vi "Append To Dataset 1D Double.vi"(8 "Error in (no error)":errorcluster, 10 "data":dbl[](array[numeric]), 11 "Dataset id in":i32) -> (0 "Error out":errorcluster, 3 "Dataset id out":i32)   [LabVIEW 2011]
uses:
  Release/HDF5Tools.dll
  HDF5Tools.lvlib
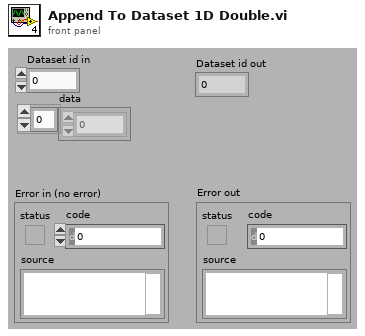
[diagram p1: front panel]
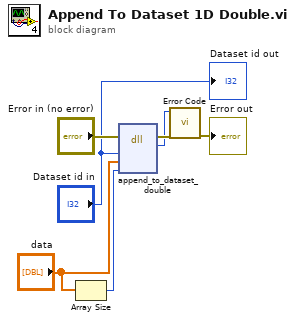
[diagram p0: block diagram]
diagram:
  n1 = Array Size(array="data") -> (size(s)=w2:i32)
  n2 = dll-call lib="F:/HDF5Tools/Release/HDF5Tools.dll" fn="append_to_dataset_double"(error in="Error in (no error)", "dataset_id"="Dataset id in", "data"="data", "count"=w2) -> (error out=w6:errorcluster, "error"=w4:i32)  [unwired: 5 in, 1 out]
  n3 = call "Error Code.vi"("Error in"=w6, "Error code"=w4) -> ("Error out"=→"Error out":errorcluster)  [unwired: 9 in]
  "Dataset id out" <- "Dataset id in"
